vi "niusrprios Scale IQ Data.vi"(0 "raw waveform data":u32[](array[numeric]), 5 "scaling (V/code)":dbl) -> (4 "scaled data":cdb[](array[numeric]))   [LabVIEW 2015]
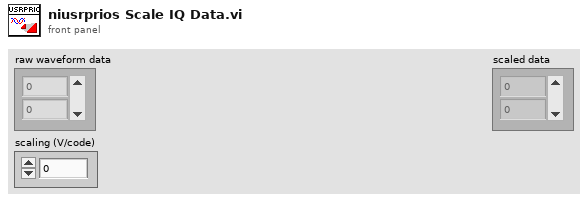
[diagram p1: front panel]
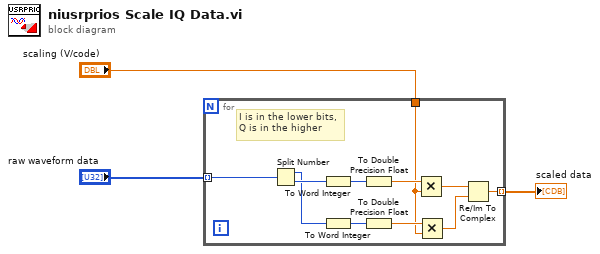
[diagram p0: block diagram]
diagram:
  n1 = for {
    tunnel: [w14] -> w2 mode=indexing
    tunnel: "raw waveform data" -> [w13] mode=indexing
    tunnel: "scaling (V/code)" -> [w4]
    # "I is in the lower bits,\nQ is in the higher"
    n2 = Split Number(x=w13) -> (hi(x)=w9:u16, lo(x)=w10:u16)
    n3 = To Word Integer(number=w10) -> (16bit integer=w8:i16)
    n4 = To Word Integer(number=w9) -> (16bit integer=w6:i16)
    n5 = To Double Precision Float(number=w8) -> (double precision float=w7:dbl)
    n6 = To Double Precision Float(number=w6) -> (double precision float=w5:dbl)
    n7 = Multiply(x=w7, y=w4) -> (x*y=w12:dbl)
    n8 = Multiply(x=w5, y=w4) -> (x*y=w11:dbl)
    n9 = Re/Im To Complex(1:w11, 2:w12) -> (0:w14:cdb)
  }
  "scaled data" <- w2
